vi "Load XML.vi"(8 "error in":errorcluster, 11 "XML Editor GUI in":refnum<class "XML Editor GUI.lvclass">) -> (0 "error out":errorcluster, 3 "XML Editor GUI out":refnum<class "XML Editor GUI.lvclass">)   [LabVIEW 2014, in "XML Editor GUI.lvclass"]
uses:
  XML Editor GUI.lvclass
  XML Document_class/XML Document.lvclass
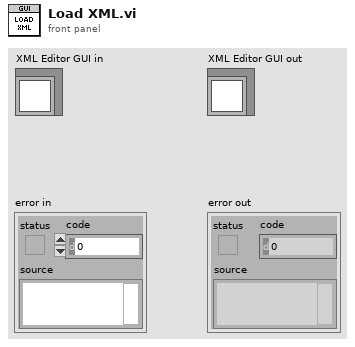
[diagram p1: front panel]
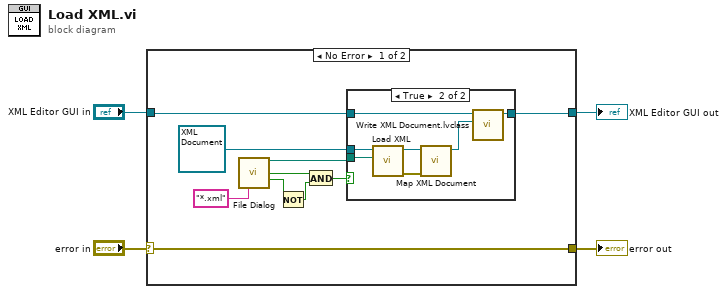
[diagram p0: block diagram]
diagram:
  n1 = case shown="No Error" "error in" {
    selector: "error in" -> [w14 w24]
    tunnel: [w14 w24] -> w3
    tunnel: [w10 w23] -> w1
    tunnel: "XML Editor GUI in" -> [w11 w23]
    frame No Error {
      n2 = call "File Dialog"("pattern (all files)"="*.xml") -> ("selected path"=w5:path, "exists"=w7:bool, "cancelled"=w8:bool)  [unwired: 11 in, 1 out]
      n3 = Not(x=w8) -> (.not. x?=w6:bool)
      n4 = And(x=w7, y=w6) -> (x .and. y?=w9:bool)
      n5 = case shown="True" w9 {
        tunnel: refnum<class "XML Document.lvclass"> refnum ("XML Document.lvclass") -> [_ w22]
        tunnel: w5 -> [_ w21]
        tunnel: [w15 w17] -> w10
        tunnel: w11 -> [w15 w16]
        frame False {
        }
        frame True {
          n6 = call "Load XML.vi"("path to XML document"=w21, "XML Document in"=w22) -> ("error out"=w19:errorcluster, "XML Document out"=w20:refnum<class "XML Document.lvclass">)  [unwired: 8 in]
          n7 = call "Map XML Document.vi"("error in"=w19, "XML Document in"=w20) -> ("XML Document out"=w18:refnum<class "XML Document.lvclass">)  [unwired: 8 in, 1 out]
          n8 = call-dynamic "Write XML Document.lvclass.vi"("XML Document.lvclass"=w18, "XML Editor GUI in"=w16) -> ("XML Editor GUI out"=w17:refnum<class "XML Editor GUI.lvclass">)  [unwired: 8 in, 1 out]
        }
      }
    }
    frame Error {
    }
  }
  "error out" <- w3
  "XML Editor GUI out" <- w1
